vi "Common-InitListBox.vi"(11 "列表框":refnum<vi>) -> ()   [LabVIEW 2014]
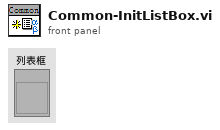
[diagram p1: front panel]
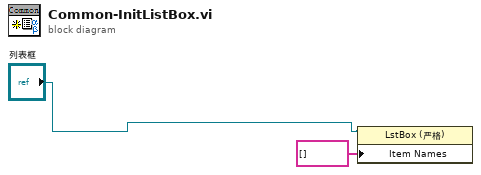
[diagram p0: block diagram]
diagram:
  n1 = property class="LstBox (严格)"(reference="列表框", "Item Names"=string[] [] ("项名")) -> ()  [unwired: 1 in, 2 out]
